vi "Enable Command Prompt.vi"(8 "error in (no error)":errorcluster, 10 "Enable Command Prompt?":bool, 11 "EPU452 in":refnum<class "EPU452.lvclass">) -> (0 "error out":errorcluster, 2 "Response":string, 3 "EPU452 out":refnum<class "EPU452.lvclass">)   [LabVIEW 2018, in "EPU452.lvclass"]
uses:
  EPU452.lvclass
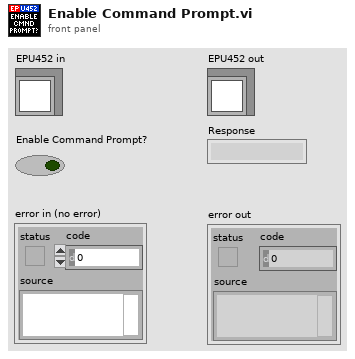
[diagram p1: front panel]
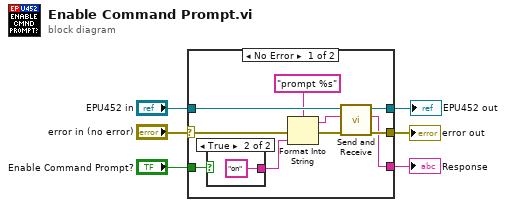
[diagram p0: block diagram]
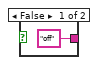
[diagram p2: hidden frame]
diagram:
  n1 = case shown="No Error" "error in (no error)" {
    selector: "error in (no error)" -> [w13 w20]
    tunnel: [w11 w20] -> w5
    tunnel: [w10 w19] -> w3
    tunnel: "EPU452 in" -> [w16 w19]
    tunnel: "Enable Command Prompt?" -> [w9 _]
    tunnel: [w7 _] -> w1
    frame No Error {
      n2 = case shown="True" w9 {
        tunnel: ["off" "on"] -> w8
        frame False {
        }
        frame True {
        }
      }
      n3 = Format Into String(format string="prompt %s", error in=w13, w8) -> (resulting string=w14:string, error out=w15:errorcluster)  [unwired: 1 in]
      n4 = call "Send and Receive.vi"("error in (no error)"=w15, "Command"=w14, "EPU452 in"=w16) -> ("error out"=w11:errorcluster, "Response"=w7:string, "EPU452 out"=w10:refnum<class "EPU452.lvclass">)  [unwired: 6 in]
    }
    frame Error {
    }
  }
  "error out" <- w5
  "EPU452 out" <- w3
  "Response" <- w1
